vi "Hysteresis RT.vi"(6 "Hysteresis [V] (1)":sgl=1.0, 8 "Threshold [V] (7)":sgl=7.0, 11 "Switch [V]":sgl) -> (3 "State":bool)   [LabVIEW 2016, in "DSI-RT.lvlib"]
uses:
  DSI-RT.lvlib
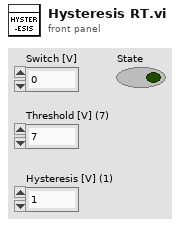
[diagram p1: front panel]
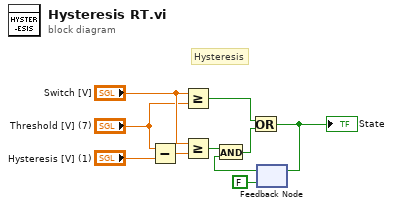
[diagram p0: block diagram]
diagram:
  # "Hysteresis"
  n1 = Subtract(x="Threshold [V] (7)", y="Hysteresis [V] (1)") -> (x-y=w8:sgl)
  n2 = Greater Or Equal?(x="Switch [V]", y="Threshold [V] (7)") -> (x >= y?=w3:bool)
  n3 = Greater Or Equal?(x="Switch [V]", y=w8) -> (x >= y?=w6:bool)
  n4 = feedback #1(FALSE) -> (w5:bool)
  n5 = And(x=w6, y=w5) -> (x .and. y?=w4:bool)
  n6 = Or(x=w3, y=w4) -> (x .or. y?=w2:bool)
  "State" <- w2
  n7 = feedback-in #1(w2) -> ()
